vi "main.vi"() -> ()   [LabVIEW 2023]
uses:
  #typedef_action.ctl
  <vilib>/Array/Sort 2D Array - Pop Stack.vi
  <vilib>/Array/Sort 2D Array - Push Stack.vi
panel:
  out "Database":string[][](array[string])
  in  "Action":T1
  in  "Nationality":string
  in  "Surname":string
  in  "Age":string
  in  "Name":string
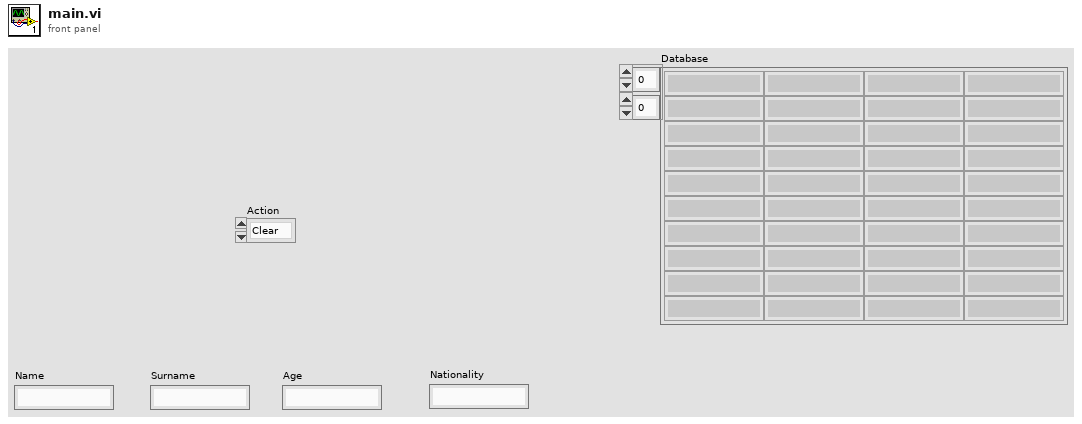
[diagram p1: front panel]
types:
  T1 = typedef "#typedef_action.ctl" = enum16{"Clear", "Add", "Sort"}
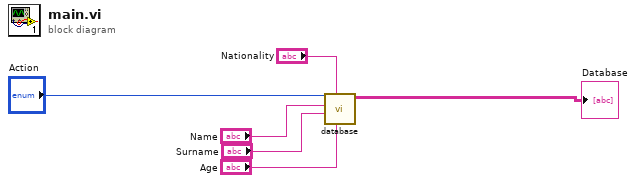
[diagram p0: block diagram]
diagram:
  n1 = call "database.vi"("Age"="Age", "Nationality"="Nationality", "Surname"="Surname", "Name"="Name", "Action"="Action") -> ("sorted 2D array"=→"Database":string[][])  [unwired: 6 in]
